vi "exec.vi"(8 "error in (no error)":errorcluster, 10 "context":refnum<class "Context.lvclass">, 11 "StartAutomatedTest in":refnum<class "StartAutomatedTest.lvclass">) -> (0 "error out":errorcluster, 2 "context 2":refnum<class "Context.lvclass">, 3 "StartAutomatedTest out":refnum<class "StartAutomatedTest.lvclass">)   [LabVIEW 2013, in "StartAutomatedTest.lvclass"]
uses:
  StartAutomatedTest.lvclass
  Context/Context.lvclass
  StartAutomatedTest.lvclass/StartAutomatedTest.ctl
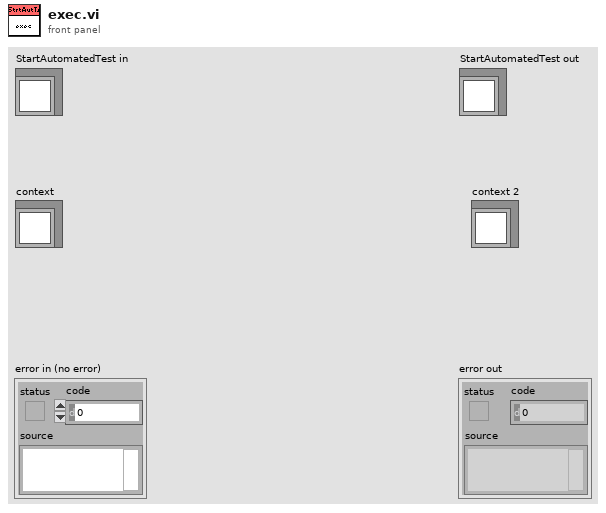
[diagram p1: front panel]
types:
  T1 = typedef "Test Parameters.ctl" = cluster{"Number of cycles for complete test":u32, "Cycle profile":T2, "Comment":string}
  T2 = typedef "CycleProfileConfig.ctl" = cluster{"Force Setpoint":dbl[unit][], "Pause After":dbl[unit][]}
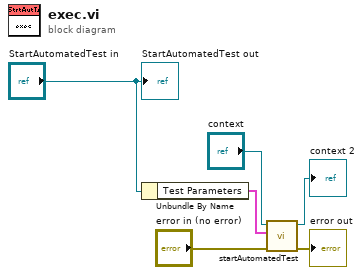
[diagram p0: block diagram]
diagram:
  n1 = Unbundle By Name("StartAutomatedTest in") -> ("Test Parameters"=w1:T1)
  n2 = call "startAutomatedTest.vi"("error in (no error)"="error in (no error)", "Test Parameters"=w1, "Context in"="context") -> ("error out"=→"error out":errorcluster, "Context out"=→"context 2":refnum<class "Context.lvclass">)  [unwired: 7 in]
  "StartAutomatedTest out" <- "StartAutomatedTest in"
